vi "SonarV7_DRONE_RT.vi"() -> ()   [LabVIEW 2017]
uses:
  <vilib>/rvi/interface/nirviReadWriteControl/nirviReadWriteControl.xnode
  <vilib>/rvi/interface/nirviCloseFPGA/nirviCloseFPGA.xnode
  <vilib>/rvi/interface/nirviOpenFPGA/nirviOpenFPGA.xnode
  <vilib>/FPGAPlugInAG/Dynamic/niLvFpga_Close_Dynamic.vi
  FPGA Bitfiles/sbRIOtest_FPGATarget2_DAQgenV4_XQOf0PBP2YY.lvbitx
  DAQgenV4.vi
  <vilib>/rvi/interface/Simulation/niFpgaSimulationCallBeginRW.vi
  <vilib>/rvi/errors/niLvFpgaAdjustHostInterfaceError.vi
panel:
  out "Elapsed Time (s)":dbl
  in  "Fs Input (Hz)":dbl=100000.0 format="%#_6p"
  in  "Fs Output (Hz)":dbl=40000.0 format="%#_6p"
  in  "Iterations":i32=25
  in  "VISA resource name":refnum<visa-resource-name>="ASRL1::INSTR"
  out "?":string
  in  "Interpulse Time (ms)":u32=1300
  in  "?":bool
  in  "Chirp Length (ms)":i32=5
  out "Echo":dbl[][](graph)
  in  "Samples to Read":i32=4000
  out "Wave Output":dbl[](graph)=[0.5, 0.5001220703125, 0.50048828125, 0.5010986328125, 0.501953125, 0.5029296875, 0.504150390625, 0.50537109375, 0.5064697265625, 0.50732421875, 0.5078125, 0.50732421875, 0.505859375, 0.5030517578125, 0.4986572265625, 0.4925537109375, 0.48486328125, 0.47607421875, 0.466796875, 0.4583740234375, 0.4522705078125, 0.4501953125, 0.4539794921875, 0.4647216796875, 0.4830322265625, 0.5078125, 0.5364990234375, 0.564697265625, 0.5865478515625, 0.5960693359375, 0.5880126953125, 0.56005859375, 0.51416015625, 0.4578857421875, 0.4039306640625, 0.3671875, 0.362060546875, 0.395751953125, 0.46533203125, 0.55419921875, 0.6357421875, 0.6796875, 0.6634521484375, 0.5838623046875, 0.463134765625, 0.345458984375, 0.2823486328125, 0.309814453125, 0.4273681640625, 0.5899658203125, 0.7216796875, 0.750244140625, 0.647705078125, 0.455810546875, 0.2747802734375, 0.213623046875, 0.32275390625, 0.5509033203125, 0.760986328125, 0.8094482421875, 0.6470947265625, 0.3704833984375, 0.1728515625, 0.2109375, 0.4754638671875, 0.7733154296875, 0.862060546875, 0.650146484375, 0.298583984375, 0.10986328125, 0.26806640625, 0.6494140625, 0.9031982421875, 0.7716064453125, 0.362548828125, 0.0799560546875, 0.2296142578125, 0.675048828125, 0.94189453125, 0.7196044921875, 0.238525390625, 0.0513916015625, 0.3975830078125, 0.877685546875, 0.8968505859375, 0.410400390625, 0.0303955078125, 0.2659912109375, 0.822265625, 0.94384765625, 0.4442138671875, 0.0172119140625, 0.28759765625, 0.8759765625, 0.9034423828125, 0.3118896484375, 0.0091552734375, 0.483642578125, 0.9871826171875, 0.6937255859375, 0.076171875, 0.17529296875, 0.8331298828125, 0.90869140625, 0.259033203125, 0.044921875, 0.663330078125, 0.975830078125, 0.391357421875, 0.0184326171875, 0.5802001953125, 0.979248046875, 0.4212646484375, 0.0286865234375, 0.6031494140625, 0.9560546875, 0.348388671875, 0.072509765625, 0.71923828125, 0.8770751953125, 0.2025146484375, 0.2047119140625, 0.87158203125, 0.6761474609375, 0.0802001953125, 0.477783203125, 0.9163818359375, 0.351318359375, 0.1612548828125, 0.8004150390625, 0.6805419921875, 0.1173095703125, 0.532958984375, 0.8494873046875, 0.2613525390625, 0.312255859375, 0.8492431640625, 0.446044921875, 0.2041015625, 0.7640380859375, 0.5853271484375, 0.1837158203125, 0.6695556640625, 0.660888671875, 0.2047119140625, 0.603271484375, 0.686279296875, 0.2335205078125, 0.573974609375, 0.6785888671875, 0.2564697265625, 0.5772705078125, 0.6473388671875, 0.274658203125, 0.603515625, 0.595458984375, 0.2991943359375, 0.6385498046875, 0.52490234375, 0.344482421875, 0.6614990234375, 0.446533203125, 0.4193115234375, 0.648193359375, 0.385986328125, 0.5128173828125, 0.5849609375, 0.37744140625, 0.587158203125, 0.4908447265625, 0.43603515625, 0.595458984375, 0.42333984375, 0.524658203125, 0.53076171875, 0.435302734375, 0.566650390625, 0.458251953125, 0.5052490234375, 0.52685546875, 0.4564208984375, 0.5426025390625, 0.471923828125, 0.5081787109375, 0.509765625, 0.479248046875, 0.5234375, 0.4805908203125, 0.51171875, 0.4964599609375, 0.4971923828125, 0.50634765625, 0.492919921875, 0.5059814453125, 0.4959716796875, 0.5020751953125, 0.499267578125, 0.5, 0.5001220703125, 0.4998779296875]
  in  "Initial Frequency (Hz)":dbl=20000.0
  in  "Final Frequency (Hz)":dbl=100000.0
  in  "Amplitude":dbl=2.0
  # "Echo-Pulse Sonar V6"
  # "To access the data, go to your web browser and type ftp://169.254.32.143/ni-rt/startup/"
  # "Wave Maker"
  # "Adding:\n-Digital signal trigger outputs to Pi\n-Sending data via serial to the Pi"
  # "Logger"
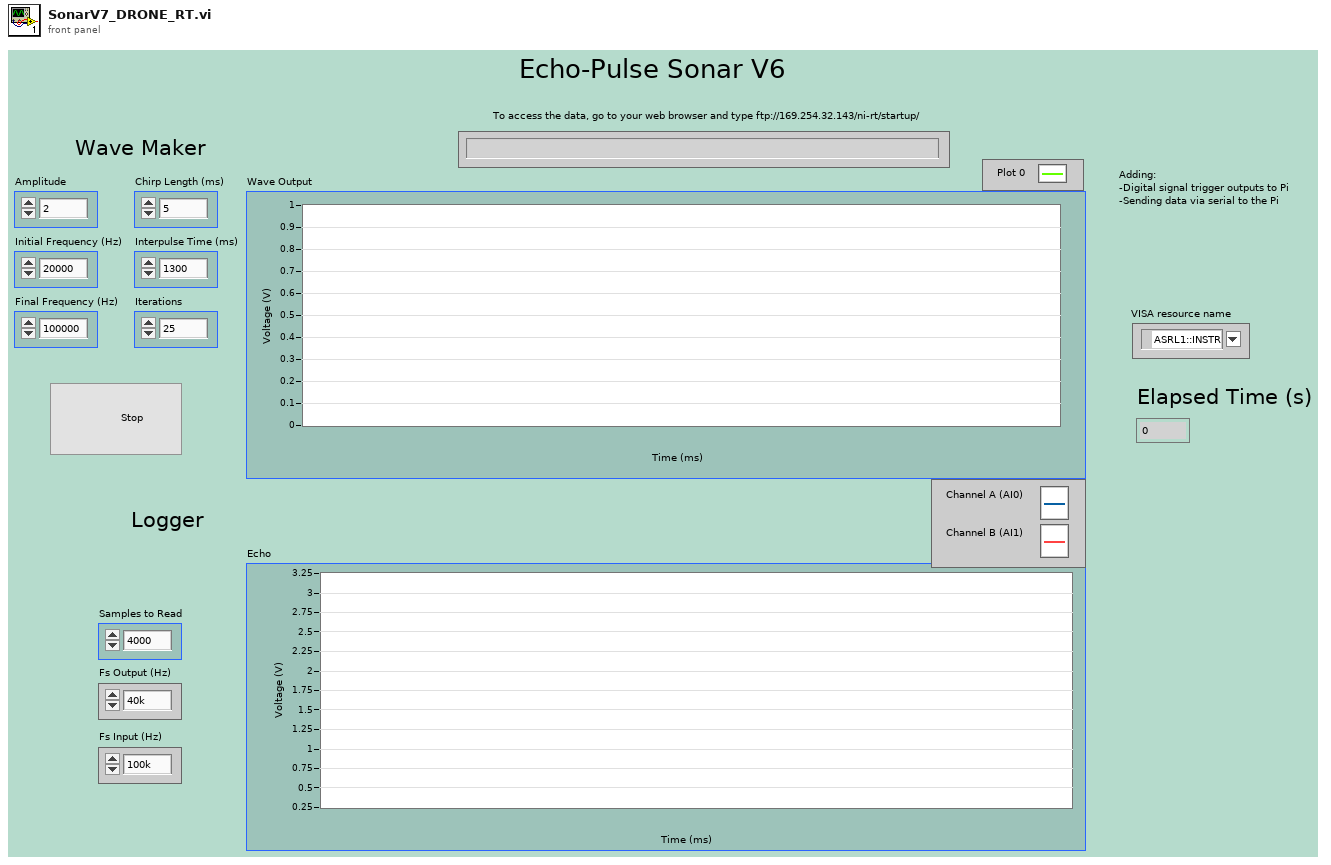
[diagram p1: front panel]
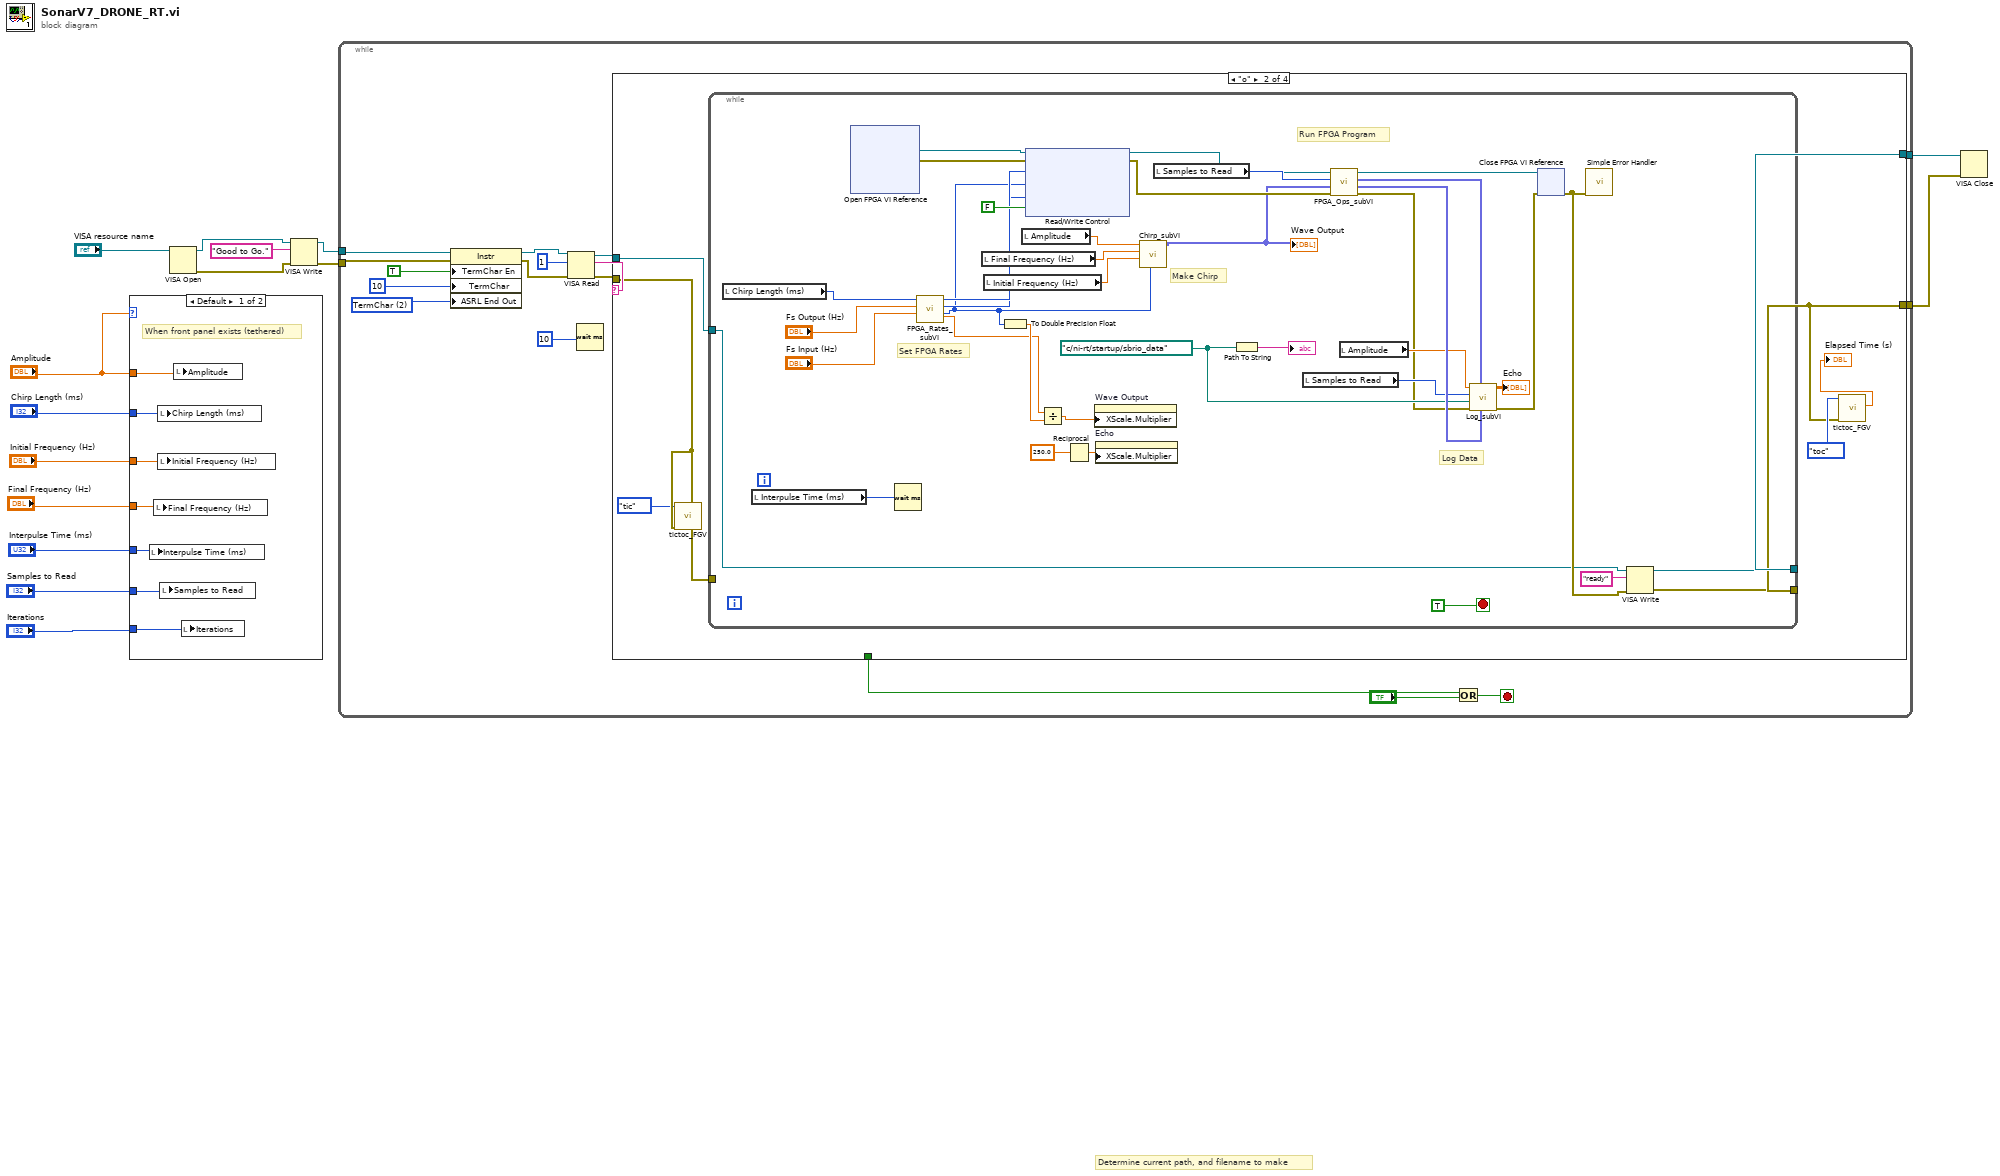
[diagram p0: block diagram]
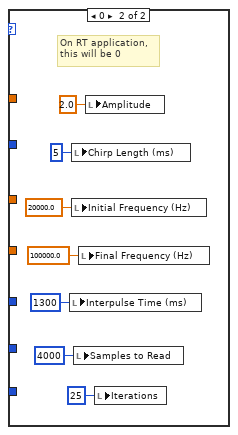
[diagram p2: hidden frame]
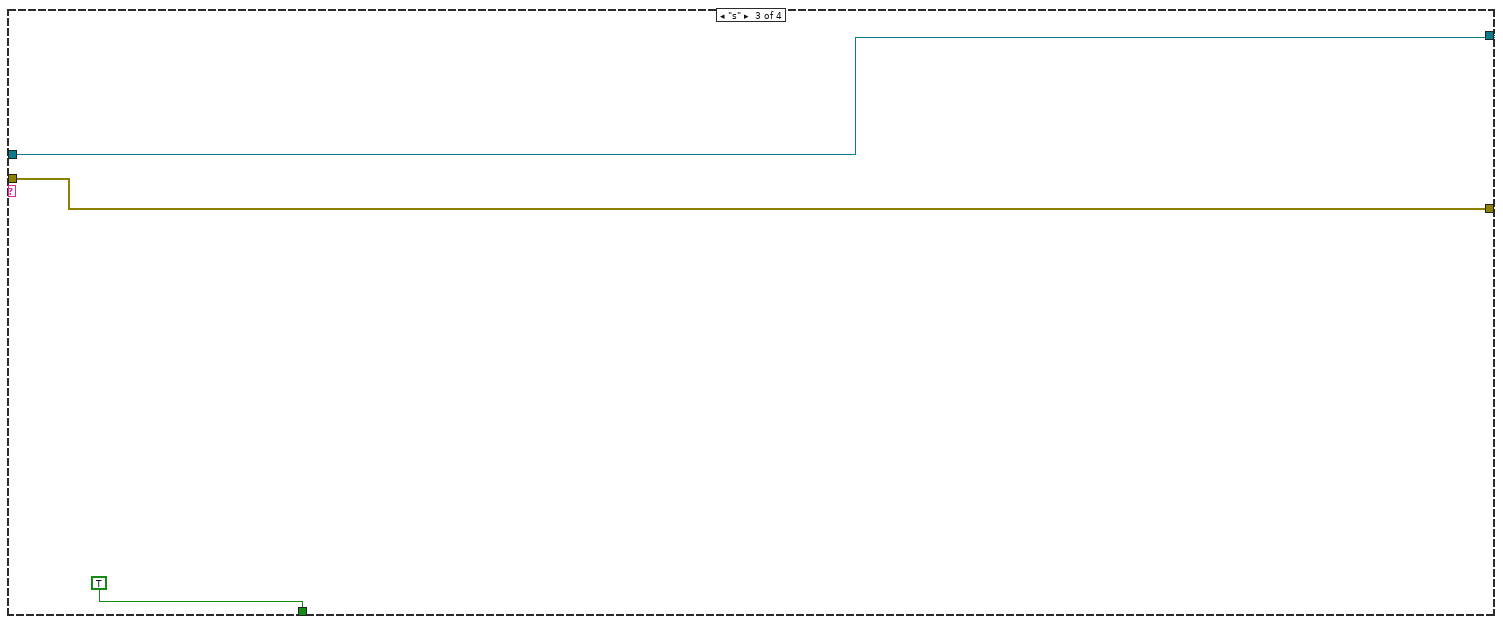
[diagram p4: hidden frame]
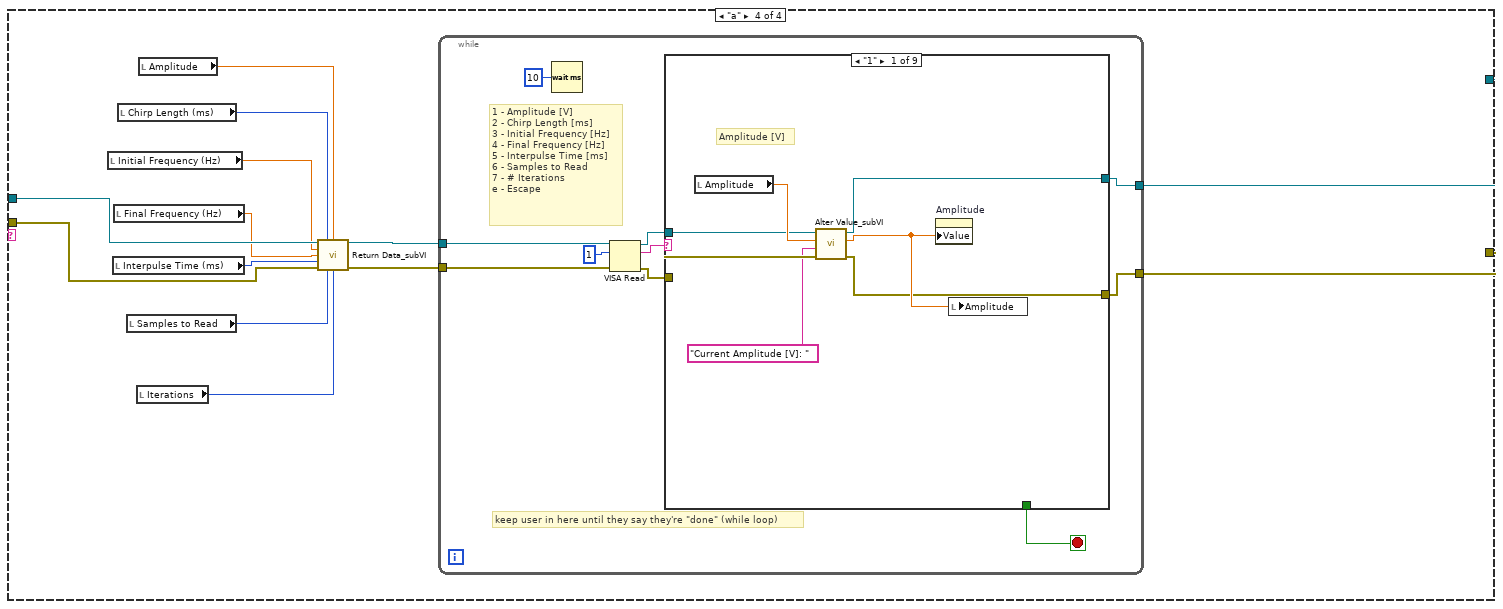
[diagram p5: hidden frame]
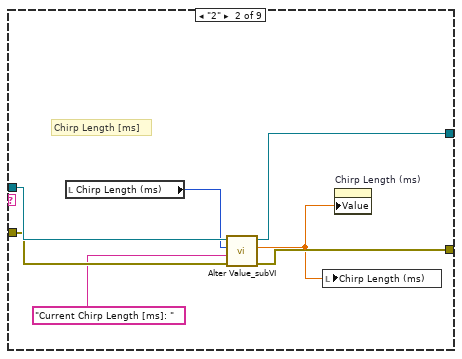
[diagram p6: hidden frame]
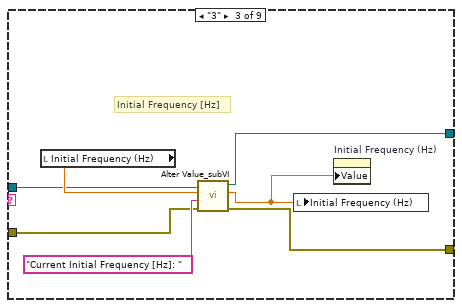
[diagram p7: hidden frame]
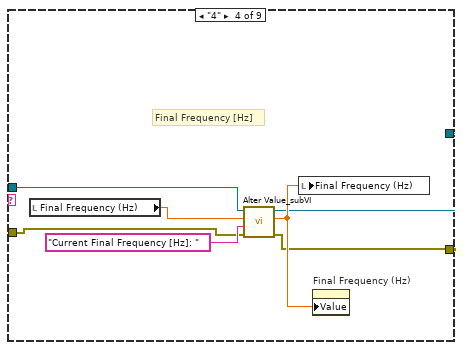
[diagram p8: hidden frame]
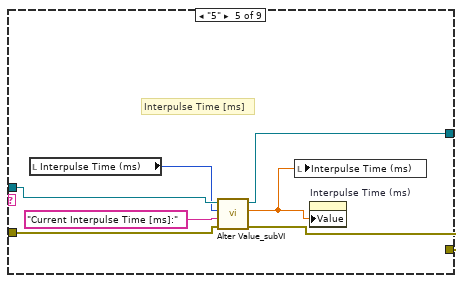
[diagram p9: hidden frame]
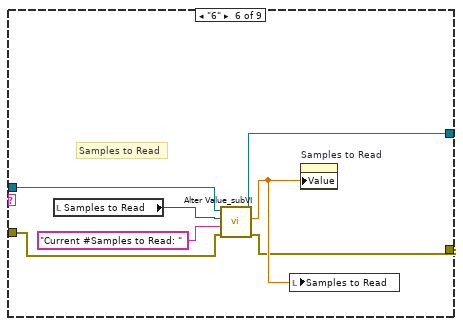
[diagram p10: hidden frame]
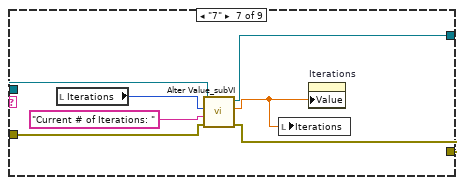
[diagram p11: hidden frame]
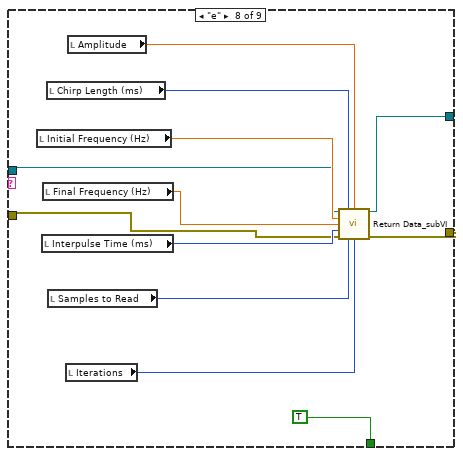
[diagram p12: hidden frame]
diagram:
  # "Determine current path, and filename to make"
  n1 = case shown="Default" "Amplitude" {
    tunnel: "Amplitude" -> [w22 _]
    tunnel: "Chirp Length (ms)" -> [w21 _]
    tunnel: "Initial Frequency (Hz)" -> [w20 _]
    tunnel: "Final Frequency (Hz)" -> [w19 _]
    tunnel: "Interpulse Time (ms)" -> [w18 _]
    tunnel: "Samples to Read" -> [w17 _]
    tunnel: "Iterations" -> [w16 _]
    frame Default {
      # "When front panel exists (tethered)"
      n2 = local write "Interpulse Time (ms)"(w18) -> ()
      n3 = local write "Final Frequency (Hz)"(w19) -> ()
      n4 = local write "Chirp Length (ms)"(w21) -> ()
      n5 = local write "Initial Frequency (Hz)"(w20) -> ()
      n6 = local write "Samples to Read"(w17) -> ()
      n7 = local write "Amplitude"(w22) -> ()
      n8 = local write "Iterations"(w16) -> ()
    }
    frame 0 {
      # "On RT application,\nthis will be 0"
      n9 = local write "Interpulse Time (ms)"(u32 1300 ("Interpulse Time (ms)")) -> ()
      n10 = local write "Chirp Length (ms)"(5 ("Chirp Length (ms)")) -> ()
      n11 = local write "Initial Frequency (Hz)"(20000.0 ("Initial Frequency (Hz)")) -> ()
      n12 = local write "Samples to Read"(4000 ("Samples to Read")) -> ()
      n13 = local write "Final Frequency (Hz)"(100000.0 ("Final Frequency (Hz)")) -> ()
      n14 = local write "Amplitude"(2.0 ("Amplitude")) -> ()
      n15 = local write "Iterations"(25 ("Iterations")) -> ()
    }
  }
  n16 = VISA Open(VISA resource name="VISA resource name") -> (VISA resource name=w14:refnum<visa-resource-name>, error out=w13:errorcluster)  [unwired: 4 in]
  n17 = VISA Write(VISA resource name=w14, write buffer="Good to Go.", error in (no error)=w13) -> (VISA resource name out=w11:refnum<visa-resource-name>, error out=w10:errorcluster)  [unwired: 1 out]
  n18 = while {
    tunnel: [w43] -> w2
    tunnel: [w42] -> w1
    tunnel: w11 -> [w35]
    tunnel: w10 -> [w34]
    stop <- w39 stop-if-true
    w36 = u16 2 items=["None", "Last Bit", "TermChar", "Break"] ("Serial Settings:End Mode for Writes")
    n19 = property class="Instr"(reference=w35, error in=w34, "TermChar En"=TRUE ("Message Based Settings:Termination Character Enable"), "TermChar"=u8 10 ("Message Based Settings:Termination Character"), "ASRL End Out"=w36) -> (reference out=w31:refnum<visa-resource-name>, error out=w30:errorcluster)
    n20 = VISA Read(VISA resource name=w31, byte count=u32 1, error in (no error)=w30) -> (VISA resource name out=w45:refnum<visa-resource-name>, read buffer=w40:string, error out=w44:errorcluster)  [unwired: 1 out]
    n21 = Wait (ms)(milliseconds to wait=u32 10) -> ()  [unwired: 1 out]
    n22 = case shown="\"o\"" w40 {
      tunnel: w45 -> [w48 w55 w95 w105]
      tunnel: w44 -> [w47 w50 w94 w97]
      tunnel: [w48 w54 w95 w107] -> w43
      tunnel: [w47 w51 w94 w106] -> w42
      tunnel: [_ _ TRUE _] -> w32
      frame "False", Default {
      }
      frame "o" {
        n23 = call "tictoc_FGV.vi"("Error In"=w50, "Case"=enum16{"tic", "toc"}."tic") -> ()  [unwired: 7 in, 2 out]
        n24 = while {
          tunnel: w55 -> [w68]
          tunnel: w50 -> [_]
          tunnel: [w93] -> w54
          tunnel: [w65] -> w51
          stop <- TRUE stop-if-true
          w78 = path "c:/ni-rt/startup/sbrio_data"
          # "Run FPGA Program"
          # "Make Chirp"
          # "Set FPGA Rates"
          # "Log Data"
          n25 = local read "Chirp Length (ms)"() -> (w74:i32)
          n26 = local read "Interpulse Time (ms)"() -> (w67:u32)
          n27 = xnode "Open FPGA VI Reference"() -> ("FPGA VI Reference Out"=w84:refnum<k20>, "error out"=w64:errorcluster)  [unwired: 2 in]
          n28 = Wait (ms)(milliseconds to wait=w67) -> ()  [unwired: 1 out]
          n29 = call "FPGA_Rates_subVI.vi"("Fs In (Hz)"="Fs Input (Hz)", "Fs Out (Hz)"="Fs Output (Hz)", "Chirp Len (ms)"=w74) -> ("# Output Samples"=w56:i16, "Input Ticks (ticks/S)"=w79:u32, "Output Ticks (ticks/S)"=w87:u32, "Chirp Len (ms)"=w82:dbl)  [unwired: 5 in]
          n30 = local read "Final Frequency (Hz)"() -> (w58:dbl)
          n31 = local read "Initial Frequency (Hz)"() -> (w59:dbl)
          n32 = To Double Precision Float(number=w56) -> (double precision float=w92:dbl)
          n33 = local read "Amplitude"() -> (w57:dbl)
          n34 = xnode "Read/Write Control"("FPGA VI Reference In"=w84, "error in"=w64, "Sampling Rate (Hz)"=w87, "# Samples"=w56, "Count(Ticks)"=w79, "Wavegen!"=FALSE) -> ("FPGA VI Reference Out"=w70:refnum<k20>, "error out"=w63:errorcluster)
          n35 = Divide(x=w82, y=w92) -> (x/y=w83:dbl)
          n36 = Reciprocal(x=250.0) -> (1/x=w85:dbl)
          n37 = property on="Wave Output" class="WFGraph (strict)"("XScale.Multiplier"=w83) -> ()  [unwired: 2 in, 2 out]
          n38 = property on="Echo" class="WFGraph (strict)"("XScale.Multiplier"=w85) -> ()  [unwired: 2 in, 2 out]
          n39 = call "Chirp_subVI.vi"("# Output Samples"=w56, "Initial Frequency (Hz)"=w59, "Final Frequency (Hz)"=w58, "Amplitude (V)"=w57) -> ("Chirp"=w60:fxp<+,16,3>[])  [unwired: 7 in]
          "Wave Output" <- w60
          n40 = local read "Samples to Read"() -> (w71:i32)
          n41 = Path To String(path=w78) -> (string=→"?":string)
          n42 = local read "Samples to Read"() -> (w72:i32)
          n43 = call "FPGA_Ops_subVI.vi"("error in (no error)"=w63, "Chirp"=w60, "Samples to Read"=w71, "FPGA VI Reference Out"=w70) -> ("error out"=w62:errorcluster, "Data B"=w90:fxp<+,16,3>[], "Data A"=w91:fxp<+,16,3>[], "Refnum out"=w89:refnum<k20>)  [unwired: 4 in]
          n44 = local read "Amplitude"() -> (w73:dbl)
          n45 = call "Log_subVI.vi"("Data B"=w90, "Data A"=w91, "error in (no error)"=w62, "Path"=w78, "Samples to Read"=w72, "Amplitude (V)"=w73) -> ("error out"=w61:errorcluster, "Echo"=→"Echo":dbl[][])  [unwired: 4 in]
          n46 = xnode "Close FPGA VI Reference"("FPGA VI Reference In"=w89, "error in"=w61) -> ("error out"=w80:errorcluster)
          n47 = call <vilib>:"Simple Error Handler.vi"("error in (no error)"=w80) -> ()  [unwired: 4 in, 5 out]
          n48 = VISA Write(VISA resource name=w68, write buffer="ready", error in (no error)=w80) -> (VISA resource name out=w93:refnum<visa-resource-name>, error out=w65:errorcluster)  [unwired: 1 out]
        }
        n49 = call "tictoc_FGV.vi"("Error In"=w51, "Case"=enum16{"tic", "toc"}."toc") -> ("Elapsed Time (s)"=→"Elapsed Time (s)":dbl)  [unwired: 7 in, 1 out]
      }
      frame "s" {
      }
      frame "a" {
        n50 = local read "Initial Frequency (Hz)"() -> (w102:dbl)
        n51 = local read "Interpulse Time (ms)"() -> (w100:u32)
        n52 = local read "Final Frequency (Hz)"() -> (w101:dbl)
        n53 = local read "Chirp Length (ms)"() -> (w103:i32)
        n54 = local read "Samples to Read"() -> (w99:i32)
        n55 = local read "Iterations"() -> (w98:i32)
        n56 = local read "Amplitude"() -> (w104:dbl)
        n57 = call "Return Data_subVI.vi"("VISA Refnum in"=w105, "Chirp Len (ms)"=w103, "Amplitude (V)"=w104, "Initial Freq (Hz)"=w102, "Final Freq (Hz)"=w101, "Interpulse Time (ms)"=w100, "error in (no error)"=w97, "Samples to Read"=w99, "Iterations"=w98) -> ("VISA Refnum out"=w109:refnum<visa-resource-name>, "error out"=w108:errorcluster)  [unwired: 5 in]
        n58 = while {
          tunnel: w109 -> [w119]
          tunnel: w108 -> [w118]
          tunnel: [w111] -> w107
          tunnel: [w110] -> w106
          stop <- w117 stop-if-true
          # "1 - Amplitude [V]\n2 - Chirp Length [ms]\n3 - Initial Frequency [Hz]\n4 - Final Frequency [Hz]\n5 - Interpulse Time [ms]\n6 - Samples to Read\n7 - # Iterations\ne - Escape"
          # "keep user in here until they say they're \"done\" (while loop)"
          n59 = Wait (ms)(milliseconds to wait=u32 10) -> ()  [unwired: 1 out]
          n60 = VISA Read(VISA resource name=w119, byte count=u32 1, error in (no error)=w118) -> (VISA resource name out=w114:refnum<visa-resource-name>, read buffer=w113:string, error out=w112:errorcluster)  [unwired: 1 out]
          n61 = case shown="\"1\"" w113 {
            tunnel: [_ _ _ _ _ _ _ TRUE _] -> w117
            tunnel: w114 -> [w124 w131 w138 w145 w154 w159 w165 w171 w182]
            tunnel: w112 -> [w123 w130 w137 w144 w153 w158 w164 w172 w181]
            tunnel: [w122 w133 w136 w141 w149 w156 w162 w170 w182] -> w111
            tunnel: [w121 w132 w135 w142 w150 w155 w163 w169 w181] -> w110
            frame "1" {
              # "Amplitude [V]"
              n62 = local read "Amplitude"() -> (w126:dbl)
              n63 = call "Alter Value_subVI.vi"("error in (no error)"=w123, "String Output"="Current Amplitude [V]: ", "Input"=w126, "VISA Refnum in"=w124) -> ("error out"=w121:errorcluster, "New Value"=w125:dbl, "VISA Refnum out"=w122:refnum<visa-resource-name>)  [unwired: 5 in]
              n64 = property on="Amplitude" class="DigNum (strict)"("Value"=w125) -> ()  [unwired: 2 in, 2 out]
              n65 = local write "Amplitude"(w125) -> ()
            }
            frame "2" {
              # "Chirp Length [ms]"
              n66 = local read "Chirp Length (ms)"() -> (w129:i32)
              n67 = call "Alter Value_subVI.vi"("error in (no error)"=w130, "String Output"="Current Chirp Length [ms]: ", "Input"=w129, "VISA Refnum in"=w131) -> ("error out"=w132:errorcluster, "New Value"=w128:dbl, "VISA Refnum out"=w133:refnum<visa-resource-name>)  [unwired: 5 in]
              n68 = local write "Chirp Length (ms)"(w128) -> ()
              n69 = property on="Chirp Length (ms)" class="DigNum (strict)"("Value"=w128) -> ()  [unwired: 2 in, 2 out]
            }
            frame "3" {
              # "Initial Frequency [Hz]"
              n70 = local read "Initial Frequency (Hz)"() -> (w140:dbl)
              n71 = call "Alter Value_subVI.vi"("error in (no error)"=w137, "String Output"="Current Initial Frequency [Hz]: " ("string"), "Input"=w140, "VISA Refnum in"=w138) -> ("error out"=w135:errorcluster, "New Value"=w134:dbl, "VISA Refnum out"=w136:refnum<visa-resource-name>)  [unwired: 5 in]
              n72 = local write "Initial Frequency (Hz)"(w134) -> ()
              n73 = property on="Initial Frequency (Hz)" class="DigNum (strict)"("Value"=w134) -> ()  [unwired: 2 in, 2 out]
            }
            frame "4" {
              # "Final Frequency [Hz]"
              n74 = local read "Final Frequency (Hz)"() -> (w147:dbl)
              n75 = call "Alter Value_subVI.vi"("error in (no error)"=w144, "String Output"="Current Final Frequency [Hz]: " ("string"), "Input"=w147, "VISA Refnum in"=w145) -> ("error out"=w142:errorcluster, "New Value"=w143:dbl, "VISA Refnum out"=w141:refnum<visa-resource-name>)  [unwired: 5 in]
              n76 = local write "Final Frequency (Hz)"(w143) -> ()
              n77 = property on="Final Frequency (Hz)" class="DigNum (strict)"("Value"=w143) -> ()  [unwired: 2 in, 2 out]
            }
            frame "5" {
              # "Interpulse Time [ms]"
              n78 = local read "Interpulse Time (ms)"() -> (w152:u32)
              n79 = call "Alter Value_subVI.vi"("error in (no error)"=w153, "String Output"="Current Interpulse Time [ms]:" ("string"), "Input"=w152, "VISA Refnum in"=w154) -> ("error out"=w150:errorcluster, "New Value"=w148:dbl, "VISA Refnum out"=w149:refnum<visa-resource-name>)  [unwired: 5 in]
              n80 = local write "Interpulse Time (ms)"(w148) -> ()
              n81 = property on="Interpulse Time (ms)" class="DigNum (strict)"("Value"=w148) -> ()  [unwired: 2 in, 2 out]
            }
            frame "6" {
              # "Samples to Read"
              n82 = local read "Samples to Read"() -> (w161:i32)
              n83 = call "Alter Value_subVI.vi"("error in (no error)"=w158, "String Output"="Current #Samples to Read: " ("string"), "Input"=w161, "VISA Refnum in"=w159) -> ("error out"=w155:errorcluster, "New Value"=w157:dbl, "VISA Refnum out"=w156:refnum<visa-resource-name>)  [unwired: 5 in]
              n84 = local write "Samples to Read"(w157) -> ()
              n85 = property on="Samples to Read" class="DigNum (strict)"("Value"=w157) -> ()  [unwired: 2 in, 2 out]
            }
            frame "7" {
              n86 = local read "Iterations"() -> (w166:i32)
              n87 = call "Alter Value_subVI.vi"("error in (no error)"=w164, "String Output"="Current # of Iterations: " ("string"), "Input"=w166, "VISA Refnum in"=w165) -> ("error out"=w163:errorcluster, "New Value"=w168:dbl, "VISA Refnum out"=w162:refnum<visa-resource-name>)  [unwired: 5 in]
              n88 = local write "Iterations"(w168) -> ()
              n89 = property on="Iterations" class="DigNum (strict)"("Value"=w168) -> ()  [unwired: 2 in, 2 out]
            }
            frame "e" {
              n90 = local read "Initial Frequency (Hz)"() -> (w177:dbl)
              n91 = local read "Interpulse Time (ms)"() -> (w175:u32)
              n92 = local read "Final Frequency (Hz)"() -> (w176:dbl)
              n93 = local read "Chirp Length (ms)"() -> (w178:i32)
              n94 = local read "Samples to Read"() -> (w174:i32)
              n95 = local read "Iterations"() -> (w173:i32)
              n96 = local read "Amplitude"() -> (w179:dbl)
              n97 = call "Return Data_subVI.vi"("VISA Refnum in"=w171, "Chirp Len (ms)"=w178, "Amplitude (V)"=w179, "Initial Freq (Hz)"=w177, "Final Freq (Hz)"=w176, "Interpulse Time (ms)"=w175, "error in (no error)"=w172, "Samples to Read"=w174, "Iterations"=w173) -> ("VISA Refnum out"=w170:refnum<visa-resource-name>, "error out"=w169:errorcluster)  [unwired: 5 in]
            }
            frame "", Default {
            }
          }
        }
      }
    }
    n98 = Or(x=w32, y="?") -> (x .or. y?=w39:bool)
  }
  n99 = VISA Close(VISA resource name=w2, error in (no error)=w1) -> ()  [unwired: 1 out]
